vi "Erweiterte Konfig_Dialog_ScreenShots.vi"(11 "VI-Referenz neu":refnum<vi>) -> (0 "Aktive Seiten":i32[](array[numeric]), 1 "Seitennamen":string[](array[string]), 3 "Elem Referenz":refnum<vi>)   [LabVIEW 2020, in "Backup.lvlib"]
uses:
  Backup.lvlib
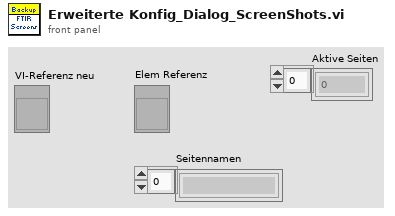
[diagram p1: front panel]
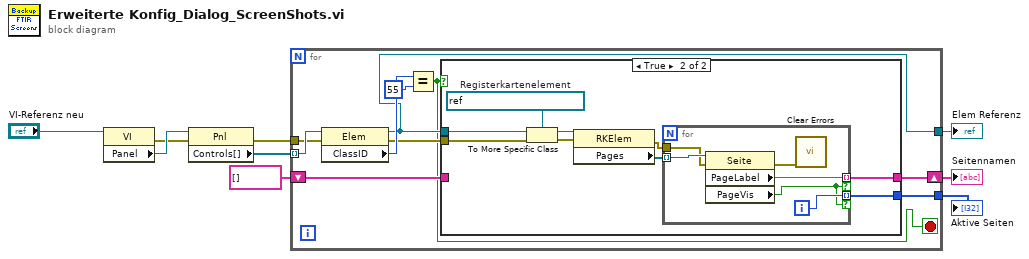
[diagram p0: block diagram]
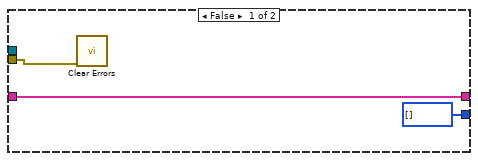
[diagram p2: hidden frame]
diagram:
  n1 = property class="VI"(reference="VI-Referenz neu") -> (error out=w6:errorcluster, "Panel"=w9:refnum<vi>)  [unwired: 1 in, 1 out]
  n2 = property class="Pnl"(reference=w9, error in=w6) -> (error out=w7:errorcluster, "Controls[]"=w5:refnum<vi>[])  [unwired: 1 out]
  n3 = for {
    tunnel: w5 -> [w17] mode=indexing
    tunnel: w7 -> [w15]
    shift-right: [w14] -> w3
    shift-left: string[] [] -> [w13]
    tunnel: [w12] -> w2
    tunnel: [w10] -> w1
    stop <- w11 stop-if-true
    n4 = property class="Elem"(reference=w17, error in=w15) -> (reference out=w12:refnum<vi>, error out=w16:errorcluster, "ClassID"=w19:u32)
    n5 = Equal?(x=w19, y=u32 55) -> (x = y?=w11:bool)
    n6 = case shown="True" w11 {
      tunnel: w12 -> [_ w31]
      tunnel: w16 -> [w22 w28]
      tunnel: [w21 w24] -> w14
      tunnel: w13 -> [w21 _]
      tunnel: [i32[] [] w23] -> w10
      frame False {
        n7 = call <vilib>:"Clear Errors.vi"("error in (no error)"=w22) -> ()  [unwired: 5 in, 2 out]
      }
      frame True {
        w29 = refnum<vi> refnum  # Registerkartenelement
        n8 = To More Specific Class(target class=w29, reference=w31, error in=w28) -> (specific class reference=w30:refnum<vi>, error out=w27:errorcluster)
        n9 = property class="RKElem"(reference=w30, error in=w27) -> (error out=w25:errorcluster, "Pages"=w26:refnum<vi>[])  [unwired: 1 out]
        n10 = for {
          tunnel: w26 -> [w37] mode=indexing
          tunnel: w25 -> [w36]
          tunnel: [w34] -> w24 mode=indexing if=w32
          tunnel: [w33] -> w23 mode=indexing if=w32
          i -> [w33]
          n11 = property class="Seite"(reference=w37, error in=w36) -> (error out=w35:errorcluster, "PageLabel"=w34:string, "PageVis"=w32:bool)  [unwired: 1 out]
          n12 = call <vilib>:"Clear Errors.vi"("error in (no error)"=w35) -> ()  [unwired: 5 in, 2 out]
        }
      }
    }
  }
  "Seitennamen" <- w3
  "Elem Referenz" <- w2
  "Aktive Seiten" <- w1
